vi "DAC Init Results.vi"(8 "error in":errorcluster, 9 "Log Details?":bool, 10 "tdms file":refnum<k34>, 11 "DAC HTS dU in":refnum<class "DAC HTS dU.lvclass">) -> (0 "error out":errorcluster, 2 "tdms file out":refnum<k34>)   [LabVIEW 2019, in "DAC.lvlib" / "DAC HTS dU.lvclass"]
uses:
  DAC HTS dU.lvclass
  DAC.lvclass
  C:/Users/wg/Documents/LV_Projects/test-stand/App/DAC/DAC.lvclass
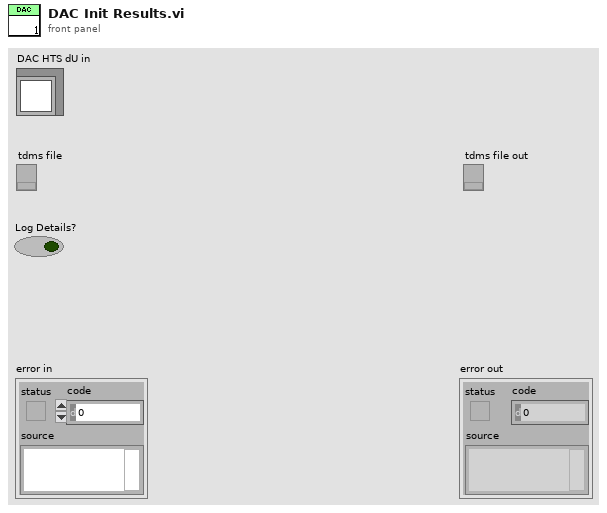
[diagram p1: front panel]
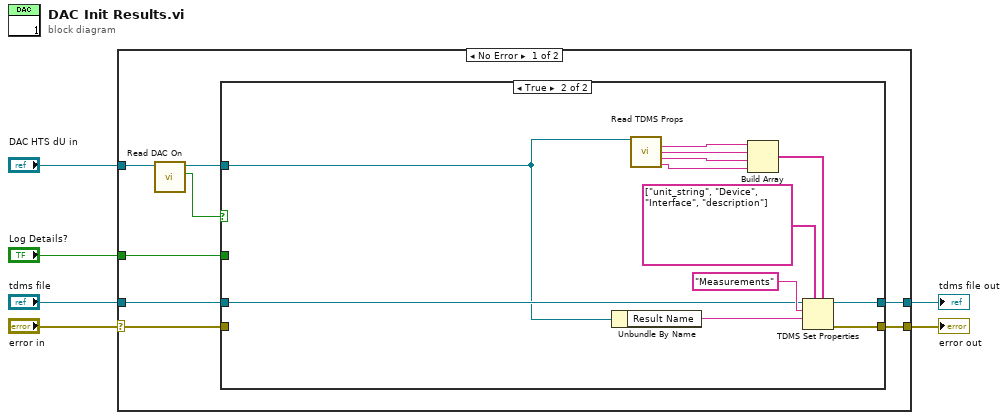
[diagram p0: block diagram]
diagram:
  n1 = case shown="No Error" "error in" {
    selector: "error in" -> [w10 w30]
    tunnel: [w7 w30] -> w6
    tunnel: "DAC HTS dU in" -> [w14 _]
    tunnel: "tdms file" -> [w11 w29]
    tunnel: [w8 w29] -> w5
    tunnel: "Log Details?" -> [w9 _]
    frame No Error {
      n2 = call "Read DAC On.vi"("DAC in"=w14) -> ("DAC On"=w12:bool, "DAC out"=w13:refnum<class "DAC HTS dU.lvclass">)  [unwired: 8 in, 1 out]
      n3 = case shown="True" w12 {
        tunnel: w11 -> [w15 w26]
        tunnel: [w15 w24] -> w8
        tunnel: [w16 w25] -> w7
        tunnel: w13 -> [_ w17]
        tunnel: w10 -> [w16 _]
        tunnel: w9 -> [_ _]
        frame False {
        }
        frame True {
          n4 = Unbundle By Name(w17) -> ("Result Name"=w27:string)
          n5 = call "Read TDMS Props.vi"("DAC in"=w17) -> ("Result Unit"=w23:string, "DAC Device"=w22:string, "DAC IO"=w21:string, "DAC Description"=w20:string)  [unwired: 10 in, 1 out]
          n6 = Build Array(w23, w22, w21, w20) -> (w18:string[])
          n7 = TDMS Set Properties(5:w18, 7:string[] ["unit_string", "Device", "Interface", "description"] ("property names"), 9:w27, 10:"Measurements" ("group name in (Untitled)"), 11:w26) -> (0:w25:errorcluster, 3:w24:refnum<k34>)  [unwired: 1 in, 2 out]
        }
      }
    }
    frame Error {
    }
  }
  "error out" <- w6
  "tdms file out" <- w5
